vi "FipsAdjacent.vi"() -> (11 "Fips":i32[](array[numeric]))   [LabVIEW 2017] (continued)
GA\"\t13185\t\"Echols County, GA\"\t13101\n\"Lowndes County, GA\"\t13185\t\"Lanier County, GA\"\t13173\n\"Lowndes County, GA\"\t13185\t\"Lowndes County, GA\"\t13185\n\"Lumpkin County, GA\"\t13187\t\"Dawson County, GA\"\t13085\n\"Lumpkin County, GA\"\t13187\t\"Fannin County, GA\"\t13111\n\"Lumpkin County, GA\"\t13187\t\"Hall County, GA\"\t13139\n\"Lumpkin County, GA\"\t13187\t\"Lumpkin County, GA\"\t13187\n\"Lumpkin County, GA\"\t13187\t\"Union County, GA\"\t13291\n\"Lumpkin County, GA\"\t13187\t\"White County, GA\"\t13311\n\"McDuffie County, GA\"\t13189\t\"Columbia County, GA\"\t13073\n\"McDuffie County, GA\"\t13189\t\"Jefferson County, GA\"\t13163\n\"McDuffie County, GA\"\t13189\t\"Lincoln County, GA\"\t13181\n\"McDuffie County, GA\"\t13189\t\"McDuffie County, GA\"\t13189\n\"McDuffie County, GA\"\t13189\t\"Richmond County, GA\"\t13245\n\"McDuffie County, GA\"\t13189\t\"Warren County, GA\"\t13301\n\"McDuffie County, GA\"\t13189\t\"Wilkes County, GA\"\t13317\n\"McIntosh County, GA\"\t13191\t\"Glynn County, GA\"\t13127\n\"McIntosh County, GA\"\t13191\t\"Liberty County, GA\"\t13179\n\"McIntosh County, GA\"\t13191\t\"Long County, GA\"\t13183\n\"McIntosh County, GA\"\t13191\t\"McIntosh County, GA\"\t13191\n\"McIntosh County, GA\"\t13191\t\"Wayne County, GA\"\t13305\n\"Macon County, GA\"\t13193\t\"Crawford County, GA\"\t13079\n\"Macon County, GA\"\t13193\t\"Dooly County, GA\"\t13093\n\"Macon County, GA\"\t13193\t\"Houston County, GA\"\t13153\n\"Macon County, GA\"\t13193\t\"Macon County, GA\"\t13193\n\"Macon County, GA\"\t13193\t\"Peach County, GA\"\t13225\n\"Macon County, GA\"\t13193\t\"Schley County, GA\"\t13249\n\"Macon County, GA\"\t13193\t\"Sumter County, GA\"\t13261\n\"Macon County, GA\"\t13193\t\"Taylor County, GA\"\t13269\n\"Madison County, GA\"\t13195\t\"Banks County, GA\"\t13011\n\"Madison County, GA\"\t13195\t\"Clarke County, GA\"\t13059\n\"Madison County, GA\"\t13195\t\"Elbert County, GA\"\t13105\n\"Madison County, GA\"\t13195\t\"Franklin County, GA\"\t13119\n\"Madison County, GA\"\t13195\t\"Hart County, GA\"\t13147\n\"Madison County, GA\"\t13195\t\"Jackson County, GA\"\t13157\n\"Madison County, GA\"\t13195\t\"Madison County, GA\"\t13195\n\"Madison County, GA\"\t13195\t\"Oglethorpe County, GA\"\t13221\n\"Marion County, GA\"\t13197\t\"Chattahoochee County, GA\"\t13053\n\"Marion County, GA\"\t13197\t\"Marion County, GA\"\t13197\n\"Marion County, GA\"\t13197\t\"Schley County, GA\"\t13249\n\"Marion County, GA\"\t13197\t\"Stewart County, GA\"\t13259\n\"Marion County, GA\"\t13197\t\"Sumter County, GA\"\t13261\n\"Marion County, GA\"\t13197\t\"Talbot County, GA\"\t13263\n\"Marion County, GA\"\t13197\t\"Taylor County, GA\"\t13269\n\"Marion County, GA\"\t13197\t\"Webster County, GA\"\t13307\n\"Meriwether County, GA\"\t13199\t\"Coweta County, GA\"\t13077\n\"Meriwether County, GA\"\t13199\t\"Harris County, GA\"\t13145\n\"Meriwether County, GA\"\t13199\t\"Meriwether County, GA\"\t13199\n\"Meriwether County, GA\"\t13199\t\"Pike County, GA\"\t13231\n\"Meriwether County, GA\"\t13199\t\"Spalding County, GA\"\t13255\n\"Meriwether County, GA\"\t13199\t\"Talbot County, GA\"\t13263\n\"Meriwether County, GA\"\t13199\t\"Troup County, GA\"\t13285\n\"Meriwether County, GA\"\t13199\t\"Upson County, GA\"\t13293\n\"Miller County, GA\"\t13201\t\"Baker County, GA\"\t13007\n\"Miller County, GA\"\t13201\t\"Decatur County, GA\"\t13087\n\"Miller County, GA\"\t13201\t\"Early County, GA\"\t13099\n\"Miller County, GA\"\t13201\t\"Miller County, GA\"\t13201\n\"Miller County, GA\"\t13201\t\"Seminole County, GA\"\t13253\n\"Mitchell County, GA\"\t13205\t\"Baker County, GA\"\t13007\n\"Mitchell County, GA\"\t13205\t\"Colquitt County, GA\"\t13071\n\"Mitchell County, GA\"\t13205\t\"Decatur County, GA\"\t13087\n\"Mitchell County, GA\"\t13205\t\"Dougherty County, GA\"\t13095\n\"Mitchell County, GA\"\t13205\t\"Grady County, GA\"\t13131\n\"Mitchell County, GA\"\t13205\t\"Mitchell County, GA\"\t13205\n\"Mitchell County, GA\"\t13205\t\"Thomas County, GA\"\t13275\n\"Mitchell County, GA\"\t13205\t\"Worth County, GA\"\t13321\n\"Monroe County, GA\"\t13207\t\"Bibb County, GA\"\t13021\n\"Monroe County, GA\"\t13207\t\"Butts County, GA\"\t13035\n\"Monroe County, GA\"\t13207\t\"Crawford County, GA\"\t13079\n\"Monroe County, GA\"\t13207\t\"Jasper County, GA\"\t13159\n\"Monroe County, GA\"\t13207\t\"Jones County, GA\"\t13169\n\"Monroe County, GA\"\t13207\t\"Lamar County, GA\"\t13171\n\"Monroe County, GA\"\t13207\t\"Monroe County, GA\"\t13207\n\"Monroe County, GA\"\t13207\t\"Upson County, GA\"\t13293\n\"Montgomery County, GA\"\t13209\t\"Jeff Davis County, GA\"\t13161\n\"Montgomery County, GA\"\t13209\t\"Montgomery County, GA\"\t13209\n\"Montgomery County, GA\"\t13209\t\"Toombs County, GA\"\t13279\n\"Montgomery County, GA\"\t13209\t\"Treutlen County, GA\"\t13283\n\"Montgomery County, GA\"\t13209\t\"Wheeler County, GA\"\t13309\n\"Morgan County, GA\"\t13211\t\"Greene County, GA\"\t13133\n\"Morgan County, GA\"\t13211\t\"Jasper County, GA\"\t13159\n\"Morgan County, GA\"\t13211\t\"Morgan County, GA\"\t13211\n\"Morgan County, GA\"\t13211\t\"Newton County, GA\"\t13217\n\"Morgan County, GA\"\t13211\t\"Oconee County, GA\"\t13219\n\"Morgan County, GA\"\t13211\t\"Putnam County, GA\"\t13237\n\"Morgan County, GA\"\t13211\t\"Walton County, GA\"\t13297\n\"Murray County, GA\"\t13213\t\"Fannin County, GA\"\t13111\n\"Murray County, GA\"\t13213\t\"Gilmer County, GA\"\t13123\n\"Murray County, GA\"\t13213\t\"Gordon County, GA\"\t13129\n\"Murray County, GA\"\t13213\t\"Murray County, GA\"\t13213\n\"Murray County, GA\"\t13213\t\"Whitfield County, GA\"\t13313\n\"Murray County, GA\"\t13213\t\"Bradley County, TN\"\t47011\n\"Murray County, GA\"\t13213\t\"Polk County, TN\"\t47139\n\"Muscogee County, GA\"\t13215\t\"Lee County, AL\"\t01081\n\"Muscogee County, GA\"\t13215\t\"Russell County, AL\"\t01113\n\"Muscogee County, GA\"\t13215\t\"Chattahoochee County, GA\"\t13053\n\"Muscogee County, GA\"\t13215\t\"Harris County, GA\"\t13145\n\"Muscogee County, GA\"\t13215\t\"Muscogee County, GA\"\t13215\n\"Muscogee County, GA\"\t13215\t\"Talbot County, GA\"\t13263\n\"Newton County, GA\"\t13217\t\"Butts County, GA\"\t13035\n\"Newton County, GA\"\t13217\t\"Henry County, GA\"\t13151\n\"Newton County, GA\"\t13217\t\"Jasper County, GA\"\t13159\n\"Newton County, GA\"\t13217\t\"Morgan County, GA\"\t13211\n\"Newton County, GA\"\t13217\t\"Newton County, GA\"\t13217\n\"Newton County, GA\"\t13217\t\"Rockdale County, GA\"\t13247\n\"Newton County, GA\"\t13217\t\"Walton County, GA\"\t13297\n\"Oconee County, GA\"\t13219\t\"Barrow County, GA\"\t13013\n\"Oconee County, GA\"\t13219\t\"Clarke County, GA\"\t13059\n\"Oconee County, GA\"\t13219\t\"Greene County, GA\"\t13133\n\"Oconee County, GA\"\t13219\t\"Jackson County, GA\"\t13157\n\"Oconee County, GA\"\t13219\t\"Morgan County, GA\"\t13211\n\"Oconee County, GA\"\t13219\t\"Oconee County, GA\"\t13219\n\"Oconee County, GA\"\t13219\t\"Oglethorpe County, GA\"\t13221\n\"Oconee County, GA\"\t13219\t\"Walton County, GA\"\t13297\n\"Oglethorpe County, GA\"\t13221\t\"Clarke County, GA\"\t13059\n\"Oglethorpe County, GA\"\t13221\t\"Elbert County, GA\"\t13105\n\"Oglethorpe County, GA\"\t13221\t\"Greene County, GA\"\t13133\n\"Oglethorpe County, GA\"\t13221\t\"Madison County, GA\"\t13195\n\"Oglethorpe County, GA\"\t13221\t\"Oconee County, GA\"\t13219\n\"Oglethorpe County, GA\"\t13221\t\"Oglethorpe County, GA\"\t13221\n\"Oglethorpe County, GA\"\t13221\t\"Taliaferro County, GA\"\t13265\n\"Oglethorpe County, GA\"\t13221\t\"Wilkes County, GA\"\t13317\n\"Paulding County, GA\"\t13223\t\"Bartow County, GA\"\t13015\n\"Paulding County, GA\"\t13223\t\"Carroll County, GA\"\t13045\n\"Paulding County, GA\"\t13223\t\"Cobb County, GA\"\t13067\n\"Paulding County, GA\"\t13223\t\"Douglas County, GA\"\t13097\n\"Paulding County, GA\"\t13223\t\"Haralson County, GA\"\t13143\n\"Paulding County, GA\"\t13223\t\"Paulding County, GA\"\t13223\n\"Paulding County, GA\"\t13223\t\"Polk County, GA\"\t13233\n\"Peach County, GA\"\t13225\t\"Crawford County, GA\"\t13079\n\"Peach County, GA\"\t13225\t\"Houston County, GA\"\t13153\n\"Peach County, GA\"\t13225\t\"Macon County, GA\"\t13193\n\"Peach County, GA\"\t13225\t\"Peach County, GA\"\t13225\n\"Peach County, GA\"\t13225\t\"Taylor County, GA\"\t13269\n\"Pickens County, GA\"\t13227\t\"Bartow County, GA\"\t13015\n\"Pickens County, GA\"\t13227\t\"Cherokee County, GA\"\t13057\n\"Pickens County, GA\"\t13227\t\"Dawson County, GA\"\t13085\n\"Pickens County, GA\"\t13227\t\"Gilmer County, GA\"\t13123\n\"Pickens County, GA\"\t13227\t\"Gordon County, GA\"\t13129\n\"Pickens County, GA\"\t13227\t\"Pickens County, GA\"\t13227\n\"Pierce County, GA\"\t13229\t\"Appling County, GA\"\t13001\n\"Pierce County, GA\"\t13229\t\"Bacon County, GA\"\t13005\n\"Pierce County, GA\"\t13229\t\"Brantley County, GA\"\t13025\n\"Pierce County, GA\"\t13229\t\"Pierce County, GA\"\t13229\n\"Pierce County, GA\"\t13229\t\"Ware County, GA\"\t13299\n\"Pierce County, GA\"\t13229\t\"Wayne County, GA\"\t13305\n\"Pike County, GA\"\t13231\t\"Lamar County, GA\"\t13171\n\"Pike County, GA\"\t13231\t\"Meriwether County, GA\"\t13199\n\"Pike County, GA\"\t13231\t\"Pike County, GA\"\t13231\n\"Pike County, GA\"\t13231\t\"Spalding County, GA\"\t13255\n\"Pike County, GA\"\t13231\t\"Upson County, GA\"\t13293\n\"Polk County, GA\"\t13233\t\"Cherokee County, AL\"\t01019\n\"Polk County, GA\"\t13233\t\"Cleburne County, AL\"\t01029\n\"Polk County, GA\"\t13233\t\"Bartow County, GA\"\t13015\n\"Polk County, GA\"\t13233\t\"Floyd County, GA\"\t13115\n\"Polk County, GA\"\t13233\t\"Haralson County, GA\"\t13143\n\"Polk County, GA\"\t13233\t\"Paulding County, GA\"\t13223\n\"Polk County, GA\"\t13233\t\"Polk County, GA\"\t13233\n\"Pulaski County, GA\"\t13235\t\"Bleckley County, GA\"\t13023\n\"Pulaski County, GA\"\t13235\t\"Dodge County, GA\"\t13091\n\"Pulaski County, GA\"\t13235\t\"Dooly County, GA\"\t13093\n\"Pulaski County, GA\"\t13235\t\"Houston County, GA\"\t13153\n\"Pulaski County, GA\"\t13235\t\"Pulaski County, GA\"\t13235\n\"Pulaski County, GA\"\t13235\t\"Wilcox County, GA\"\t13315\n\"Putnam County, GA\"\t13237\t\"Baldwin County, GA\"\t13009\n\"Putnam County, GA\"\t13237\t\"Greene County, GA\"\t13133\n\"Putnam County, GA\"\t13237\t\"Hancock County, GA\"\t13141\n\"Putnam County, GA\"\t13237\t\"Jasper County, GA\"\t13159\n\"Putnam County, GA\"\t13237\t\"Jones County, GA\"\t13169\n\"Putnam County, GA\"\t13237\t\"Morgan County, GA\"\t13211\n\"Putnam County, GA\"\t13237\t\"Putnam County, GA\"\t13237\n\"Quitman County, GA\"\t13239\t\"Barbour County, AL\"\t01005\n\"Quitman County, GA\"\t13239\t\"Clay County, GA\"\t13061\n\"Quitman County, GA\"\t13239\t\"Quitman County, GA\"\t13239\n\"Quitman County, GA\"\t13239\t\"Randolph County, GA\"\t13243\n\"Quitman County, GA\"\t13239\t\"Stewart County, GA\"\t13259\n\"Rabun County, GA\"\t13241\t\"Habersham County, GA\"\t13137\n\"Rabun County, GA\"\t13241\t\"Rabun County, GA\"\t13241\n\"Rabun County, GA\"\t13241\t\"Towns County, GA\"\t13281\n\"Rabun County, GA\"\t13241\t\"Clay County, NC\"\t37043\n\"Rabun County, GA\"\t13241\t\"Jackson County, NC\"\t37099\n\"Rabun County, GA\"\t13241\t\"Macon County, NC\"\t37113\n\"Rabun County, GA\"\t13241\t\"Oconee County, SC\"\t45073\n\"Randolph County, GA\"\t13243\t\"Calhoun County, GA\"\t13037\n\"Randolph County, GA\"\t13243\t\"Clay County, GA\"\t13061\n\"Randolph County, GA\"\t13243\t\"Quitman County, GA\"\t13239\n\"Randolph County, GA\"\t13243\t\"Randolph County, GA\"\t13243\n\"Randolph County, GA\"\t13243\t\"Stewart County, GA\"\t13259\n\"Randolph County, GA\"\t13243\t\"Terrell County, GA\"\t13273\n\"Randolph County, GA\"\t13243\t\"Webster County, GA\"\t13307\n\"Richmond County, GA\"\t13245\t\"Burke County, GA\"\t13033\n\"Richmond County, GA\"\t13245\t\"Columbia County, GA\"\t13073\n\"Richmond County, GA\"\t13245\t\"Jefferson County, GA\"\t13163\n\"Richmond County, GA\"\t13245\t\"McDuffie County, GA\"\t13189\n\"Richmond County, GA\"\t13245\t\"Richmond County, GA\"\t13245\n\"Richmond County, GA\"\t13245\t\"Aiken County, SC\"\t45003\n\"Richmond County, GA\"\t13245\t\"Edgefield County, SC\"\t45037\n\"Rockdale County, GA\"\t13247\t\"DeKalb County, GA\"\t13089\n\"Rockdale County, GA\"\t13247\t\"Gwinnett County, GA\"\t13135\n\"Rockdale County, GA\"\t13247\t\"Henry County, GA\"\t13151\n\"Rockdale County, GA\"\t13247\t\"Newton County, GA\"\t13217\n\"Rockdale County, GA\"\t13247\t\"Rockdale County, GA\"\t13247\n\"Rockdale County, GA\"\t13247\t\"Walton County, GA\"\t13297\n\"Schley County, GA\"\t13249\t\"Macon County, GA\"\t13193\n\"Schley County, GA\"\t13249\t\"Marion County, GA\"\t13197\n\"Schley County, GA\"\t13249\t\"Schley County, GA\"\t13249\n\"Schley County, GA\"\t13249\t\"Sumter County, GA\"\t13261\n\"Schley County, GA\"\t13249\t\"Taylor County, GA\"\t13269\n\"Screven County, GA\"\t13251\t\"Bulloch County, GA\"\t13031\n\"Screven County, GA\"\t13251\t\"Burke County, GA\"\t13033\n\"Screven County, GA\"\t13251\t\"Effingham County, GA\"\t13103\n\"Screven County, GA\"\t13251\t\"Jenkins County, GA\"\t13165\n\"Screven County, GA\"\t13251\t\"Screven County, GA\"\t13251\n\"Screven County, GA\"\t13251\t\"Allendale County, SC\"\t45005\n\"Screven County, GA\"\t13251\t\"Hampton County, SC\"\t45049\n\"Seminole County, GA\"\t13253\t\"Houston County, AL\"\t01069\n\"Seminole County, GA\"\t13253\t\"Gadsden County, FL\"\t12039\n\"Seminole County, GA\"\t13253\t\"Jackson County, FL\"\t12063\n\"Seminole County, GA\"\t13253\t\"Decatur County, GA\"\t13087\n\"Seminole County, GA\"\t13253\t\"Early County, GA\"\t13099\n\"Seminole County, GA\"\t13253\t\"Miller County, GA\"\t13201\n\"Seminole County, GA\"\t13253\t\"Seminole County, GA\"\t13253\n\"Spalding County, GA\"\t13255\t\"Butts County, GA\"\t13035\n\"Spalding County, GA\"\t13255\t\"Clayton County, GA\"\t13063\n\"Spalding County, GA\"\t13255\t\"Coweta County, GA\"\t13077\n\"Spalding County, GA\"\t13255\t\"Fayette County, GA\"\t13113\n\"Spalding County, GA\"\t13255\t\"Henry County, GA\"\t13151\n\"Spalding County, GA\"\t13255\t\"Lamar County, GA\"\t13171\n\"Spalding County, GA\"\t13255\t\"Meriwether County, GA\"\t13199\n\"Spalding County, GA\"\t13255\t\"Pike County, GA\"\t13231\n\"Spalding County, GA\"\t13255\t\"Spalding County, GA\"\t13255\n\"Stephens County, GA\"\t13257\t\"Banks County, GA\"\t13011\n\"Stephens County, GA\"\t13257\t\"Franklin County, GA\"\t13119\n\"Stephens County, GA\"\t13257\t\"Habersham County, GA\"\t13137\n\"Stephens County, GA\"\t13257\t\"Stephens County, GA\"\t13257\n\"Stephens County, GA\"\t13257\t\"Oconee County, SC\"\t45073\n\"Stewart County, GA\"\t13259\t\"Barbour County, AL\"\t01005\n\"Stewart County, GA\"\t13259\t\"Russell County, AL\"\t01113\n\"Stewart County, GA\"\t13259\t\"Chattahoochee County, GA\"\t13053\n\"Stewart County, GA\"\t13259\t\"Marion County, GA\"\t13197\n\"Stewart County, GA\"\t13259\t\"Quitman County, GA\"\t13239\n\"Stewart County, GA\"\t13259\t\"Randolph County, GA\"\t13243\n\"Stewart County, GA\"\t13259\t\"Stewart County, GA\"\t13259\n\"Stewart County, GA\"\t13259\t\"Webster County, GA\"\t13307\n\"Sumter County, GA\"\t13261\t\"Crisp County, GA\"\t13081\n\"Sumter County, GA\"\t13261\t\"Dooly County, GA\"\t13093\n\"Sumter County, GA\"\t13261\t\"Lee County, GA\"\t13177\n\"Sumter County, GA\"\t13261\t\"Macon County, GA\"\t13193\n\"Sumter County, GA\"\t13261\t\"Marion County, GA\"\t13197\n\"Sumter County, GA\"\t13261\t\"Schley County, GA\"\t13249\n\"Sumter County, GA\"\t13261\t\"Sumter County, GA\"\t13261\n\"Sumter County, GA\"\t13261\t\"Terrell County, GA\"\t13273\n\"Sumter County, GA\"\t13261\t\"Webster County, GA\"\t13307\n\"Talbot County, GA\"\t13263\t\"Chattahoochee County, GA\"\t13053\n\"Talbot County, GA\"\t13263\t\"Harris County, GA\"\t13145\n\"Talbot County, GA\"\t13263\t\"Marion County, GA\"\t13197\n\"Talbot County, GA\"\t13263\t\"Meriwether County, GA\"\t13199\n\"Talbot County, GA\"\t13263\t\"Muscogee County, GA\"\t13215\n\"Talbot County, GA\"\t13263\t\"Talbot County, GA\"\t13263\n\"Talbot County, GA\"\t13263\t\"Taylor County, GA\"\t13269\n\"Talbot County, GA\"\t13263\t\"Upson County, GA\"\t13293\n\"Taliaferro County, GA\"\t13265\t\"Greene County, GA\"\t13133\n\"Taliaferro County, GA\"\t13265\t\"Hancock County, GA\"\t13141\n\"Taliaferro County, GA\"\t13265\t\"Oglethorpe County, GA\"\t13221\n\"Taliaferro County, GA\"\t13265\t\"Taliaferro County, GA\"\t13265\n\"Taliaferro County, GA\"\t13265\t\"Warren County, GA\"\t13301\n\"Taliaferro County, GA\"\t13265\t\"Wilkes County, GA\"\t13317\n\"Tattnall County, GA\"\t13267\t\"Appling County, GA\"\t13001\n\"Tattnall County, GA\"\t13267\t\"Candler County, GA\"\t13043\n\"Tattnall County, GA\"\t13267\t\"Emanuel County, GA\"\t13107\n\"Tattnall County, GA\"\t13267\t\"Evans County, GA\"\t13109\n\"Tattnall County, GA\"\t13267\t\"Liberty County, GA\"\t13179\n\"Tattnall County, GA\"\t13267\t\"Long County, GA\"\t13183\n\"Tattnall County, GA\"\t13267\t\"Tattnall County, GA\"\t13267\n\"Tattnall County, GA\"\t13267\t\"Toombs County, GA\"\t13279\n\"Tattnall County, GA\"\t13267\t\"Wayne County, GA\"\t13305\n\"Taylor County, GA\"\t13269\t\"Crawford County, GA\"\t13079\n\"Taylor County, GA\"\t13269\t\"Macon County, GA\"\t13193\n\"Taylor County, GA\"\t13269\t\"Marion County, GA\"\t13197\n\"Taylor County, GA\"\t13269\t\"Peach County, GA\"\t13225\n\"Taylor County, GA\"\t13269\t\"Schley County, GA\"\t13249\n\"Taylor County, GA\"\t13269\t\"Talbot County, GA\"\t13263\n\"Taylor County, GA\"\t13269\t\"Taylor County, GA\"\t13269\n\"Taylor County, GA\"\t13269\t\"Upson County, GA\"\t13293\n\"Telfair County, GA\"\t13271\t\"Ben Hill County, GA\"\t13017\n\"Telfair County, GA\"\t13271\t\"Coffee County, GA\"\t13069\n\"Telfair County, GA\"\t13271\t\"Dodge County, GA\"\t13091\n\"Telfair County, GA\"\t13271\t\"Jeff Davis County, GA\"\t13161\n\"Telfair County, GA\"\t13271\t\"Telfair County, GA\"\t13271\n\"Telfair County, GA\"\t13271\t\"Wheeler County, GA\"\t13309\n\"Telfair County, GA\"\t13271\t\"Wilcox County, GA\"\t13315\n\"Terrell County, GA\"\t13273\t\"Calhoun County, GA\"\t13037\n\"Terrell County, GA\"\t13273\t\"Dougherty County, GA\"\t13095\n\"Terrell County, GA\"\t13273\t\"Lee County, GA\"\t13177\n\"Terrell County, GA\"\t13273\t\"Randolph County, GA\"\t13243\n\"Terrell County, GA\"\t13273\t\"Sumter County, GA\"\t13261\n\"Terrell County, GA\"\t13273\t\"Terrell County, GA\"\t13273\n\"Terrell County, GA\"\t13273\t\"Webster County, GA\"\t13307\n\"Thomas County, GA\"\t13275\t\"Jefferson County, FL\"\t12065\n\"Thomas County, GA\"\t13275\t\"Leon County, FL\"\t12073\n\"Thomas County, GA\"\t13275\t\"Brooks County, GA\"\t13027\n\"Thomas County, GA\"\t13275\t\"Colquitt County, GA\"\t13071\n\"Thomas County, GA\"\t13275\t\"Grady County, GA\"\t13131\n\"Thomas County, GA\"\t13275\t\"Mitchell County, GA\"\t13205\n\"Thomas County, GA\"\t13275\t\"Thomas County, GA\"\t13275\n\"Tift County, GA\"\t13277\t\"Berrien County, GA\"\t13019\n\"Tift County, GA\"\t13277\t\"Colquitt County, GA\"\t13071\n\"Tift County, GA\"\t13277\t\"Cook County, GA\"\t13075\n\"Tift County, GA\"\t13277\t\"Irwin County, GA\"\t13155\n\"Tift County, GA\"\t13277\t\"Tift County, GA\"\t13277\n\"Tift County, GA\"\t13277\t\"Turner County, GA\"\t13287\n\"Tift County, GA\"\t13277\t\"Worth County, GA\"\t13321\n\"Toombs County, GA\"\t13279\t\"Appling County, GA\"\t13001\n\"Toombs County, GA\"\t13279\t\"Candler County, GA\"\t13043\n\"Toombs County, GA\"\t13279\t\"Emanuel County, GA\"\t13107\n\"Toombs County, GA\"\t13279\t\"Jeff Davis County, GA\"\t13161\n\"Toombs County, GA\"\t13279\t\"Montgomery County, GA\"\t13209\n\"Toombs County, GA\"\t13279\t\"Tattnall County, GA\"\t13267\n\"Toombs County, GA\"\t13279\t\"Toombs County, GA\"\t13279\n\"Toombs County, GA\"\t13279\t\"Treutlen County, GA\"\t13283\n\"Towns County, GA\"\t13281\t\"Habersham County, GA\"\t13137\n\"Towns County, GA\"\t13281\t\"Rabun County, GA\"\t13241\n\"Towns County, GA\"\t13281\t\"Towns County, GA\"\t13281\n\"Towns County, GA\"\t13281\t\"Union County, GA\"\t13291\n\"Towns County, GA\"\t13281\t\"White County, GA\"\t13311\n\"Towns County, GA\"\t13281\t\"Clay County, NC\"\t37043\n\"Treutlen County, GA\"\t13283\t\"Emanuel County, GA\"\t13107\n\"Treutlen County, GA\"\t13283\t\"Johnson County, GA\"\t13167\n\"Treutlen County, GA\"\t13283\t\"Laurens County, GA\"\t13175\n\"Treutlen County, GA\"\t13283\t\"Montgomery County, GA\"\t13209\n\"Treutlen County, GA\"\t13283\t\"Toombs County, GA\"\t13279\n\"Treutlen County, GA\"\t13283\t\"Treutlen County, GA\"\t13283\n\"Treutlen County, GA\"\t13283\t\"Wheeler County, GA\"\t13309\n\"Troup County, GA\"\t13285\t\"Chambers County, AL\"\t01017\n\"Troup County, GA\"\t13285\t\"Randolph County, AL\"\t01111\n\"Troup County, GA\"\t13285\t\"Coweta County, GA\"\t13077\n\"Troup County, GA\"\t13285\t\"Harris County, GA\"\t13145\n\"Troup County, GA\"\t13285\t\"Heard County, GA\"\t13149\n\"Troup County, GA\"\t13285\t\"Meriwether County, GA\"\t13199\n\"Troup County, GA\"\t13285\t\"Troup County, GA\"\t13285\n\"Turner County, GA\"\t13287\t\"Ben Hill County, GA\"\t13017\n\"Turner County, GA\"\t13287\t\"Crisp County, GA\"\t13081\n\"Turner County, GA\"\t13287\t\"Irwin County, GA\"\t13155\n\"Turner County, GA\"\t13287\t\"Tift County, GA\"\t13277\n\"Turner County, GA\"\t13287\t\"Turner County, GA\"\t13287\n\"Turner County, GA\"\t13287\t\"Wilcox County, GA\"\t13315\n\"Turner County, GA\"\t13287\t\"Worth County, GA\"\t13321\n\"Twiggs County, GA\"\t13289\t\"Bibb County, GA\"\t13021\n\"Twiggs County, GA\"\t13289\t\"Bleckley County, GA\"\t13023\n\"Twiggs County, GA\"\t13289\t\"Houston County, GA\"\t13153\n\"Twiggs County, GA\"\t13289\t\"Jones County, GA\"\t13169\n\"Twiggs County, GA\"\t13289\t\"Laurens County, GA\"\t13175\n\"Twiggs County, GA\"\t13289\t\"Twiggs County, GA\"\t13289\n\"Twiggs County, GA\"\t13289\t\"Wilkinson County, GA\"\t13319\n\"Union County, GA\"\t13291\t\"Fannin County, GA\"\t13111\n\"Union County, GA\"\t13291\t\"Lumpkin County, GA\"\t13187\n\"Union County, GA\"\t13291\t\"Towns County, GA\"\t13281\n\"Union County, GA\"\t13291\t\"Union County, GA\"\t13291\n\"Union County, GA\"\t13291\t\"White County, GA\"\t13311\n\"Union County, GA\"\t13291\t\"Cherokee County, NC\"\t37039\n\"Union County, GA\"\t13291\t\"Clay County, NC\"\t37043\n\"Upson County, GA\"\t13293\t\"Crawford County, GA\"\t13079\n\"Upson County, GA\"\t13293\t\"Lamar County, GA\"\t13171\n\"Upson County, GA\"\t13293\t\"Meriwether County, GA\"\t13199\n\"Upson County, GA\"\t13293\t\"Monroe County, GA\"\t13207\n\"Upson County, GA\"\t13293\t\"Pike County, GA\"\t13231\n\"Upson County, GA\"\t13293\t\"Talbot County, GA\"\t13263\n\"Upson County, GA\"\t13293\t\"Taylor County, GA\"\t13269\n\"Upson County, GA\"\t13293\t\"Upson County, GA\"\t13293\n\"Walker County, GA\"\t13295\t\"DeKalb County, AL\"\t01049\n\"Walker County, GA\"\t13295\t\"Catoosa County, GA\"\t13047\n\"Walker County, GA\"\t13295\t\"Chattooga County, GA\"\t13055\n\"Walker County, GA\"\t13295\t\"Dade County, GA\"\t13083\n\"Walker County, GA\"\t13295\t\"Floyd County, GA\"\t13115\n\"Walker County, GA\"\t13295\t\"Gordon County, GA\"\t13129\n\"Walker County, GA\"\t13295\t\"Walker County, GA\"\t13295\n\"Walker County, GA\"\t13295\t\"Whitfield County, GA\"\t13313\n\"Walker County, GA\"\t13295\t\"Hamilton County, TN\"\t47065\n\"Walton County, GA\"\t13297\t\"Barrow County, GA\"\t13013\n\"Walton County, GA\"\t13297\t\"Gwinnett County, GA\"\t13135\n\"Walton County, GA\"\t13297\t\"Morgan County, GA\"\t13211\n\"Walton County, GA\"\t13297\t\"Newton County, GA\"\t13217\n\"Walton County, GA\"\t13297\t\"Oconee County, GA\"\t13219\n\"Walton County, GA\"\t13297\t\"Rockdale County, GA\"\t13247\n\"Walton County, GA\"\t13297\t\"Walton County, GA\"\t13297\n\"Ware County, GA\"\t13299\t\"Baker County, FL\"\t12003\n\"Ware County, GA\"\t13299\t\"Atkinson County, GA\"\t13003\n\"Ware County, GA\"\t13299\t\"Bacon County, GA\"\t13005\n\"Ware County, GA\"\t13299\t\"Brantley County, GA\"\t13025\n\"Ware County, GA\"\t13299\t\"Charlton County, GA\"\t13049\n\"Ware County, GA\"\t13299\t\"Clinch County, GA\"\t13065\n\"Ware County, GA\"\t13299\t\"Coffee County, GA\"\t13069\n\"Ware County, GA\"\t13299\t\"Pierce County, GA\"\t13229\n\"Ware County, GA\"\t13299\t\"Ware County, GA\"\t13299\n\"Warren County, GA\"\t13301\t\"Glascock County, GA\"\t13125\n\"Warren County, GA\"\t13301\t\"Hancock County, GA\"\t13141\n\"Warren County, GA\"\t13301\t\"Jefferson County, GA\"\t13163\n\"Warren County, GA\"\t13301\t\"McDuffie County, GA\"\t13189\n\"Warren County, GA\"\t13301\t\"Taliaferro County, GA\"\t13265\n\"Warren County, GA\"\t13301\t\"Warren County, GA\"\t13301\n\"Warren County, GA\"\t13301\t\"Wilkes County, GA\"\t13317\n\"Washington County, GA\"\t13303\t\"Baldwin County, GA\"\t13009\n\"Washington County, GA\"\t13303\t\"Glascock County, GA\"\t13125\n\"Washington County, GA\"\t13303\t\"Hancock County, GA\"\t13141\n\"Washington County, GA\"\t13303\t\"Jefferson County, GA\"\t13163\n\"Washington County, GA\"\t13303\t\"Johnson County, GA\"\t13167\n\"Washington County, GA\"\t13303\t\"Washington County, GA\"\t13303\n\"Washington County, GA\"\t13303\t\"Wilkinson County, GA\"\t13319\n\"Wayne County, GA\"\t13305\t\"Appling County, GA\"\t13001\n\"Wayne County, GA\"\t13305\t\"Brantley County, GA\"\t13025\n\"Wayne County, GA\"\t13305\t\"Glynn County, GA\"\t13127\n\"Wayne County, GA\"\t13305\t\"Long County, GA\"\t13183\n\"Wayne County, GA\"\t13305\t\"McIntosh County, GA\"\t13191\n\"Wayne County, GA\"\t13305\t\"Pierce County, GA\"\t13229\n\"Wayne County, GA\"\t13305\t\"Tattnall County, GA\"\t13267\n\"Wayne County, GA\"\t13305\t\"Wayne County, GA\"\t13305\n\"Webster County, GA\"\t13307\t\"Marion County, GA\"\t13197\n\"Webster County, GA\"\t13307\t\"Randolph County, GA\"\t13243\n\"Webster County, GA\"\t13307\t\"Stewart County, GA\"\t13259\n\"Webster County, GA\"\t13307\t\"Sumter County, GA\"\t13261\n\"Webster County, GA\"\t13307\t\"Terrell County, GA\"\t13273\n\"Webster County, GA\"\t13307\t\"Webster County, GA\"\t13307\n\"Wheeler County, GA\"\t13309\t\"Dodge County, GA\"\t13091\n\"Wheeler County, GA\"\t13309\t\"Jeff Davis County, GA\"\t13161\n\"Wheeler County, GA\"\t13309\t\"Laurens County, GA\"\t13175\n\"Wheeler County, GA\"\t13309\t\"Montgomery County, GA\"\t13209\n\"Wheeler County, GA\"\t13309\t\"Telfair County, GA\"\t13271\n\"Wheeler County, GA\"\t13309\t\"Treutlen County, GA\"\t13283\n\"Wheeler County, GA\"\t13309\t\"Wheeler County, GA\"\t13309\n\"White County, GA\"\t13311\t\"Habersham County, GA\"\t13137\n\"White County, GA\"\t13311\t\"Hall County, GA\"\t13139\n\"White County, GA\"\t13311\t\"Lumpkin County, GA\"\t13187\n\"White County, GA\"\t13311\t\"Towns County, GA\"\t13281\n\"White County, GA\"\t13311\t\"Union County, GA\"\t13291\n\"White County, GA\"\t13311\t\"White County, GA\"\t13311\n\"Whitfield County, GA\"\t13313\t\"Catoosa County, GA\"\t13047\n\"Whitfield County, GA\"\t13313\t\"Gordon County, GA\"\t13129\n\"Whitfield County, GA\"\t13313\t\"Murray County, GA\"\t13213\n\"Whitfield County, GA\"\t13313\t\"Walker County, GA\"\t13295\n\"Whitfield County, GA\"\t13313\t\"Whitfield County, GA\"\t13313\n\"Whitfield County, GA\"\t13313\t\"Bradley County, TN\"\t47011\n\"Whitfield County, GA\"\t13313\t\"Hamilton County, TN\"\t47065\n\"Wilcox County, GA\"\t13315\t\"Ben Hill County, GA\"\t13017\n\"Wilcox County, GA\"\t13315\t\"Crisp County, GA\"\t13081\n\"Wilcox County, GA\"\t13315\t\"Dodge County, GA\"\t13091\n\"Wilcox County, GA\"\t13315\t\"Dooly County, GA\"\t13093\n\"Wilcox County, GA\"\t13315\t\"Pulaski County, GA\"\t13235\n\"Wilcox County, GA\"\t13315\t\"Telfair County, GA\"\t13271\n\"Wilcox County, GA\"\t13315\t\"Turner County, GA\"\t13287\n\"Wilcox County, GA\"\t13315\t\"Wilcox County, GA\"\t13315\n\"Wilkes County, GA\"\t13317\t\"Elbert County, GA\"\t13105\n\"Wilkes County, GA\"\t13317\t\"Lincoln County, GA\"\t13181\n\"Wilkes County, GA\"\t13317\t\"McDuffie County, GA\"\t13189\n\"Wilkes County, GA\"\t13317\t\"Oglethorpe County, GA\"\t13221\n\"Wilkes County, GA\"\t13317\t\"Taliaferro County, GA\"\t13265\n\"Wilkes County, GA\"\t13317\t\"Warren County, GA\"\t13301\n\"Wilkes County, GA\"\t13317\t\"Wilkes County, GA\"\t13317\n\"Wilkinson County, GA\"\t13319\t\"Baldwin County, GA\"\t13009\n\"Wilkinson County, GA\"\t13319\t\"Bleckley County, GA\"\t13023\n\"Wilkinson County, GA\"\t13319\t\"Johnson County, GA\"\t13167\n\"Wilkinson County, GA\"\t13319\t\"Jones County, GA\"\t13169\n\"Wilkinson County, GA\"\t13319\t\"Laurens County, GA\"\t13175\n\"Wilkinson County, GA\"\t13319\t\"Twiggs County, GA\"\t13289\n\"Wilkinson County, GA\"\t13319\t\"Washington County, GA\"\t13303\n\"Wilkinson County, GA\"\t13319\t\"Wilkinson County, GA\"\t13319\n\"Worth County, GA\"\t13321\t\"Colquitt County, GA\"\t13071\n\"Worth County, GA\"\t13321\t\"Crisp County, GA\"\t13081\n\"Worth County, GA\"\t13321\t\"Dougherty County, GA\"\t13095\n\"Worth County, GA\"\t13321\t\"Lee County, GA\"\t13177\n\"Worth County, GA\"\t13321\t\"Mitchell County, GA\"\t13205\n\"Worth County, GA\"\t13321\t\"Tift County, GA\"\t13277\n\"Worth County, GA\"\t13321\t\"Turner County, GA\"\t13287\n\"Worth County, GA\"\t13321\t\"Worth County, GA\"\t13321\n\"Hawaii County, HI\"\t15001\t\"Hawaii County, HI\"\t15001\n\"Honolulu County, HI\"\t15003\t\"Honolulu County, HI\"\t15003\n\"Kalawao County, HI\"\t15005\t\"Kalawao County, HI\"\t15005\n\"Kalawao County, HI\"\t15005\t\"Maui County, HI\"\t15009\n\"Kauai County, HI\"\t15007\t\"Kauai County, HI\"\t15007\n\"Maui County, HI\"\t15009\t\"Kalawao County, HI\"\t15005\n\"Maui County, HI\"\t15009\t\"Maui County, HI\"\t15009\n\"Ada County, ID\"\t16001\t\"Ada County, ID\"\t16001\n\"Ada County, ID\"\t16001\t\"Boise County, ID\"\t16015\n\"Ada County, ID\"\t16001\t\"Canyon County, ID\"\t16027\n\"Ada County, ID\"\t16001\t\"Elmore County, ID\"\t16039\n\"Ada County, ID\"\t16001\t\"Gem County, ID\"\t16045\n\"Ada County, ID\"\t16001\t\"Owyhee County, ID\"\t16073\n\"Adams County, ID\"\t16003\t\"Adams County, ID\"\t16003\n\"Adams County, ID\"\t16003\t\"Gem County, ID\"\t16045\n\"Adams County, ID\"\t16003\t\"Idaho County, ID\"\t16049\n\"Adams County, ID\"\t16003\t\"Valley County, ID\"\t16085\n\"Adams County, ID\"\t16003\t\"Washington County, ID\"\t16087\n\"Adams County, ID\"\t16003\t\"Baker County, OR\"\t41001\n\"Adams County, ID\"\t16003\t\"Wallowa County, OR\"\t41063\n\"Bannock County, ID\"\t16005\t\"Bannock County, ID\"\t16005\n\"Bannock County, ID\"\t16005\t\"Bingham County, ID\"\t16011\n\"Bannock County, ID\"\t16005\t\"Caribou County, ID\"\t16029\n\"Bannock County, ID\"\t16005\t\"Franklin County, ID\"\t16041\n\"Bannock County, ID\"\t16005\t\"Oneida County, ID\"\t16071\n\"Bannock County, ID\"\t16005\t\"Power County, ID\"\t16077\n\"Bear Lake County, ID\"\t16007\t\"Bear Lake County, ID\"\t16007\n\"Bear Lake County, ID\"\t16007\t\"Caribou County, ID\"\t16029\n\"Bear Lake County, ID\"\t16007\t\"Franklin County, ID\"\t16041\n\"Bear Lake County, ID\"\t16007\t\"Cache County, UT\"\t49005\n\"Bear Lake County, ID\"\t16007\t\"Rich County, UT\"\t49033\n\"Bear Lake County, ID\"\t16007\t\"Lincoln County, WY\"\t56023\n\"Benewah County, ID\"\t16009\t\"Benewah County, ID\"\t16009\n\"Benewah County, ID\"\t16009\t\"Kootenai County, ID\"\t16055\n\"Benewah County, ID\"\t16009\t\"Latah County, ID\"\t16057\n\"Benewah County, ID\"\t16009\t\"Shoshone County, ID\"\t16079\n\"Benewah County, ID\"\t16009\t\"Spokane County, WA\"\t53063\n\"Benewah County, ID\"\t16009\t\"Whitman County, WA\"\t53075\n\"Bingham County, ID\"\t16011\t\"Bannock County, ID\"\t16005\n\"Bingham County, ID\"\t16011\t\"Bingham County, ID\"\t16011\n\"Bingham County, ID\"\t16011\t\"Blaine County, ID\"\t16013\n\"Bingham County, ID\"\t16011\t\"Bonneville County, ID\"\t16019\n\"Bingham County, ID\"\t16011\t\"Butte County, ID\"\t16023\n\"Bingham County, ID\"\t16011\t\"Caribou County, ID\"\t16029\n\"Bingham County, ID\"\t16011\t\"Jefferson County, ID\"\t16051\n\"Bingham County, ID\"\t16011\t\"Power County, ID\"\t16077\n\"Blaine County, ID\"\t16013\t\"Bingham County, ID\"\t16011\n\"Blaine County, ID\"\t16013\t\"Blaine County, ID\"\t16013\n\"Blaine County, ID\"\t16013\t\"Butte County, ID\"\t16023\n\"Blaine County, ID\"\t16013\t\"Camas County, ID\"\t16025\n\"Blaine County, ID\"\t16013\t\"Cassia County, ID\"\t16031\n\"Blaine County, ID\"\t16013\t\"Custer County, ID\"\t16037\n\"Blaine County, ID\"\t16013\t\"Elmore County, ID\"\t16039\n\"Blaine County, ID\"\t16013\t\"Lincoln County, ID\"\t16063\n\"Blaine County, ID\"\t16013\t\"Minidoka County, ID\"\t16067\n\"Blaine County, ID\"\t16013\t\"Power County, ID\"\t16077\n\"Boise County, ID\"\t16015\t\"Ada County, ID\"\t16001\n\"Boise County, ID\"\t16015\t\"Boise County, ID\"\t16015\n\"Boise County, ID\"\t16015\t\"Custer County, ID\"\t16037\n\"Boise County, ID\"\t16015\t\"Elmore County, ID\"\t16039\n\"Boise County, ID\"\t16015\t\"Gem County, ID\"\t16045\n\"Boise County, ID\"\t16015\t\"Valley County, ID\"\t16085\n\"Bonner County, ID\"\t16017\t\"Bonner County, ID\"\t16017\n\"Bonner County, ID\"\t16017\t\"Boundary County, ID\"\t16021\n\"Bonner County, ID\"\t16017\t\"Kootenai County, ID\"\t16055\n\"Bonner County, ID\"\t16017\t\"Shoshone County, ID\"\t16079\n\"Bonner County, ID\"\t16017\t\"Lincoln County, MT\"\t30053\n\"Bonner County, ID\"\t16017\t\"Sanders County, MT\"\t30089\n\"Bonner County, ID\"\t16017\t\"Pend Oreille County, WA\"\t53051\n\"Bonner County, ID\"\t16017\t\"Spokane County, WA\"\t53063\n\"Bonneville County, ID\"\t16019\t\"Bingham County, ID\"\t16011\n\"Bonneville County, ID\"\t16019\t\"Bonneville County, ID\"\t16019\n\"Bonneville County, ID\"\t16019\t\"Caribou County, ID\"\t16029\n\"Bonneville County, ID\"\t16019\t\"Jefferson County, ID\"\t16051\n\"Bonneville County, ID\"\t16019\t\"Madison County, ID\"\t16065\n\"Bonneville County, ID\"\t16019\t\"Teton County, ID\"\t16081\n\"Bonneville County, ID\"\t16019\t\"Lincoln County, WY\"\t56023\n\"Bonneville County, ID\"\t16019\t\"Teton County, WY\"\t56039\n\"Boundary County, ID\"\t16021\t\"Bonner County, ID\"\t16017\n\"Boundary County, ID\"\t16021\t\"Boundary County, ID\"\t16021\n\"Boundary County, ID\"\t16021\t\"Lincoln County, MT\"\t30053\n\"Boundary County, ID\"\t16021\t\"Pend Oreille County, WA\"\t53051\n\"Butte County, ID\"\t16023\t\"Bingham County, ID\"\t16011\n\"Butte County, ID\"\t16023\t\"Blaine County, ID\"\t16013\n\"Butte County, ID\"\t16023\t\"Butte County, ID\"\t16023\n\"Butte County, ID\"\t16023\t\"Clark County, ID\"\t16033\n\"Butte County, ID\"\t16023\t\"Custer County, ID\"\t16037\n\"Butte County, ID\"\t16023\t\"Jefferson County, ID\"\t16051\n\"Butte County, ID\"\t16023\t\"Lemhi County, ID\"\t16059\n\"Camas County, ID\"\t16025\t\"Blaine County, ID\"\t16013\n\"Camas County, ID\"\t16025\t\"Camas County, ID\"\t16025\n\"Camas County, ID\"\t16025\t\"Elmore County, ID\"\t16039\n\"Camas County, ID\"\t16025\t\"Gooding County, ID\"\t16047\n\"Camas County, ID\"\t16025\t\"Lincoln County, ID\"\t16063\n\"Canyon County, ID\"\t16027\t\"Ada County, ID\"\t16001\n\"Canyon County, ID\"\t16027\t\"Canyon County, ID\"\t16027\n\"Canyon County, ID\"\t16027\t\"Gem County, ID\"\t16045\n\"Canyon County, ID\"\t16027\t\"Owyhee County, ID\"\t16073\n\"Canyon County, ID\"\t16027\t\"Payette County, ID\"\t16075\n\"Canyon County, ID\"\t16027\t\"Malheur County, OR\"\t41045\n\"Caribou County, ID\"\t16029\t\"Bannock County, ID\"\t16005\n\"Caribou County, ID\"\t16029\t\"Bear Lake County, ID\"\t16007\n\"Caribou County, ID\"\t16029\t\"Bingham County, ID\"\t16011\n\"Caribou County, ID\"\t16029\t\"Bonneville County, ID\"\t16019\n\"Caribou County, ID\"\t16029\t\"Caribou County, ID\"\t16029\n\"Caribou County, ID\"\t16029\t\"Franklin County, ID\"\t16041\n\"Caribou County, ID\"\t16029\t\"Lincoln County, WY\"\t56023\n\"Cassia County, ID\"\t16031\t\"Blaine County, ID\"\t16013\n\"Cassia County, ID\"\t16031\t\"Cassia County, ID\"\t16031\n\"Cassia County, ID\"\t16031\t\"Jerome County, ID\"\t16053\n\"Cassia County, ID\"\t16031\t\"Minidoka County, ID\"\t16067\n\"Cassia County, ID\"\t16031\t\"Oneida County, ID\"\t16071\n\"Cassia County, ID\"\t16031\t\"Power County, ID\"\t16077\n\"Cassia County, ID\"\t16031\t\"Twin Falls County, ID\"\t16083\n\"Cassia County, ID\"\t16031\t\"Elko County, NV\"\t32007\n\"Cassia County, ID\"\t16031\t\"Box Elder County, UT\"\t49003\n\"Clark County, ID\"\t16033\t\"Butte County, ID\"\t16023\n\"Clark County, ID\"\t16033\t\"Clark County, ID\"\t16033\n\"Clark County, ID\"\t16033\t\"Fremont County, ID\"\t16043\n\"Clark County, ID\"\t16033\t\"Jefferson County, ID\"\t16051\n\"Clark County, ID\"\t16033\t\"Lemhi County, ID\"\t16059\n\"Clark County, ID\"\t16033\t\"Beaverhead County, MT\"\t30001\n\"Clearwater County, ID\"\t16035\t\"Clearwater County, ID\"\t16035\n\"Clearwater County, ID\"\t16035\t\"Idaho County, ID\"\t16049\n\"Clearwater County, ID\"\t16035\t\"Latah County, ID\"\t16057\n\"Clearwater County, ID\"\t16035\t\"Lewis County, ID\"\t16061\n\"Clearwater County, ID\"\t16035\t\"Nez Perce County, ID\"\t16069\n\"Clearwater County, ID\"\t16035\t\"Shoshone County, ID\"\t16079\n\"Clearwater County, ID\"\t16035\t\"Mineral County, MT\"\t30061\n\"Clearwater County, ID\"\t16035\t\"Missoula County, MT\"\t30063\n\"Custer County, ID\"\t16037\t\"Blaine County, ID\"\t16013\n\"Custer County, ID\"\t16037\t\"Boise County, ID\"\t16015\n\"Custer County, ID\"\t16037\t\"Butte County, ID\"\t16023\n\"Custer County, ID\"\t16037\t\"Custer County, ID\"\t16037\n\"Custer County, ID\"\t16037\t\"Elmore County, ID\"\t16039\n\"Custer County, ID\"\t16037\t\"Lemhi County, ID\"\t16059\n\"Custer County, ID\"\t16037\t\"Valley County, ID\"\t16085\n\"Elmore County, ID\"\t16039\t\"Ada County, ID\"\t16001\n\"Elmore County, ID\"\t16039\t\"Blaine County, ID\"\t16013\n\"Elmore County, ID\"\t16039\t\"Boise County, ID\"\t16015\n\"Elmore County, ID\"\t16039\t\"Camas County, ID\"\t16025\n\"Elmore County, ID\"\t16039\t\"Custer County, ID\"\t16037\n\"Elmore County, ID\"\t16039\t\"Elmore County, ID\"\t16039\n\"Elmore County, ID\"\t16039\t\"Gooding County, ID\"\t16047\n\"Elmore County, ID\"\t16039\t\"Owyhee County, ID\"\t16073\n\"Elmore County, ID\"\t16039\t\"Twin Falls County, ID\"\t16083\n\"Franklin County, ID\"\t16041\t\"Bannock County, ID\"\t16005\n\"Franklin County, ID\"\t16041\t\"Bear Lake County, ID\"\t16007\n\"Franklin County, ID\"\t16041\t\"Caribou County, ID\"\t16029\n\"Franklin County, ID\"\t16041\t\"Franklin County, ID\"\t16041\n\"Franklin County, ID\"\t16041\t\"Oneida County, ID\"\t16071\n\"Franklin County, ID\"\t16041\t\"Cache County, UT\"\t49005\n\"Franklin County, ID\"\t16041\t\"Rich County, UT\"\t49033\n\"Fremont County, ID\"\t16043\t\"Clark County, ID\"\t16033\n\"Fremont County, ID\"\t16043\t\"Fremont County, ID\"\t16043\n\"Fremont County, ID\"\t16043\t\"Jefferson County, ID\"\t16051\n\"Fremont County, ID\"\t16043\t\"Madison County, ID\"\t16065\n\"Fremont County, ID\"\t16043\t\"Teton County, ID\"\t16081\n\"Fremont County, ID\"\t16043\t\"Beaverhead County, MT\"\t30001\n\"Fremont County, ID\"\t16043\t\"Gallatin County, MT\"\t30031\n\"Fremont County, ID\"\t16043\t\"Madison County, MT\"\t30057\n\"Fremont County, ID\"\t16043\t\"Teton County, WY\"\t56039\n\"Gem County, ID\"\t16045\t\"Ada County, ID\"\t16001\n\"Gem County, ID\"\t16045\t\"Adams County, ID\"\t16003\n\"Gem County, ID\"\t16045\t\"Boise County, ID\"\t16015\n\"Gem County, ID\"\t16045\t\"Canyon County, ID\"\t16027\n\"Gem County, ID\"\t16045\t\"Gem County, ID\"\t16045\n\"Gem County, ID\"\t16045\t\"Payette County, ID\"\t16075\n\"Gem County, ID\"\t16045\t\"Valley County, ID\"\t16085\n\"Gem County, ID\"\t16045\t\"Washington County, ID\"\t16087\n\"Gooding County, ID\"\t16047\t\"Camas County, ID\"\t16025\n\"Gooding County, ID\"\t16047\t\"Elmore County, ID\"\t16039\n\"Gooding County, ID\"\t16047\t\"Gooding County, ID\"\t16047\n\"Gooding County, ID\"\t16047\t\"Jerome County, ID\"\t16053\n\"Gooding County, ID\"\t16047\t\"Lincoln County, ID\"\t16063\n\"Gooding County, ID\"\t16047\t\"Twin Falls County, ID\"\t16083\n\"Idaho County, ID\"\t16049\t\"Adams County, ID\"\t16003\n\"Idaho County, ID\"\t16049\t\"Clearwater County, ID\"\t16035\n\"Idaho County, ID\"\t16049\t\"Idaho County, ID\"\t16049\n\"Idaho County, ID\"\t16049\t\"Lemhi County, ID\"\t16059\n\"Idaho County, ID\"\t16049\t\"Lewis County, ID\"\t16061\n\"Idaho County, ID\"\t16049\t\"Nez 
